vi "Publish Sample.vi"(8 "error in (no error)":errorcluster, 9 "Sample in":refnum<class "Sample.lvclass">, 11 "Transfer Line in":refnum<class "Transfer Line.lvclass">) -> (0 "error out":errorcluster, 3 "Transfer Line out":refnum<class "Transfer Line.lvclass">)   [LabVIEW 2015, in "cRIO-Carbondioxide.lvlib" / "CO2-Actor.lvlib" / "Transfer Line.lvclass"]
uses:
  Transfer Line.lvclass
  subs/Sample/Sample.lvclass
  Transfer Line.lvclass/Transfer Line.ctl
  subs/Sample/Read Sample From Container.vi
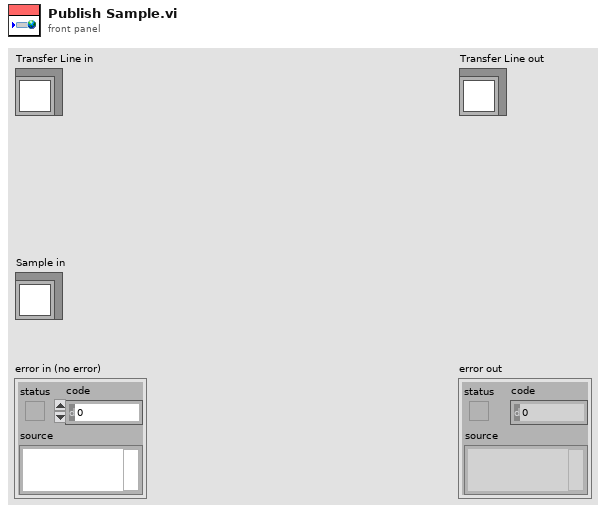
[diagram p1: front panel]
types:
  T1 = typedef "Sample Container.ctl" = cluster{"Sample In":refnum<k21>, "Sample Name":refnum<k21>, "Ti Cathode":refnum<k21>, "SampleQ":refnum<queue>}
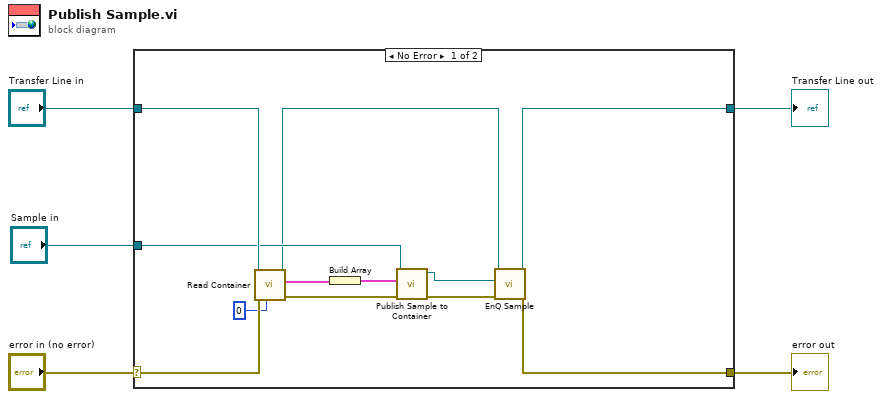
[diagram p0: block diagram]
diagram:
  n1 = case shown="No Error" "error in (no error)" {
    selector: "error in (no error)" -> [w15 w19]
    tunnel: [w10 w19] -> w4
    tunnel: [w8 w18] -> w2
    tunnel: "Transfer Line in" -> [w13 w18]
    tunnel: "Sample in" -> [w12 _]
    frame No Error {
      n2 = call "Read Container.vi"("Queue timeout in ms (-1)"=0, "error in (no error)"=w15, "Transfer Line in"=w13) -> ("error out"=w14:errorcluster, "Sample Container"=w17:T1, "Transfer Line out"=w9:refnum<class "Transfer Line.lvclass">)  [unwired: 4 in, 2 out]
      n3 = Build Array(w17) -> (w16:T1[])
      n4 = call "Publish Sample to Container.vi"("error in (no error)"=w14, "Containers"=w16, "Sample in"=w12) -> ("error out"=w11:errorcluster, "Sample out"=w7:refnum<class "Sample.lvclass">)  [unwired: 7 in]
      n5 = call "EnQ Sample.vi"("error in (no error)"=w11, "Sample.lvclass"=w7, "Transfer Line in"=w9) -> ("error out"=w10:errorcluster, "Transfer Line out"=w8:refnum<class "Transfer Line.lvclass">)  [unwired: 7 in]
    }
    frame Error {
    }
  }
  "error out" <- w4
  "Transfer Line out" <- w2
